vi "linspace_double.vi"(9 "start":dbl format="%0.2f", 10 "end":dbl=1.0 format="%0.2f", 11 "samples":dbl=128.0) -> (3 "Ramp Pattern":dbl[](array[numeric]))   [LabVIEW 2019]
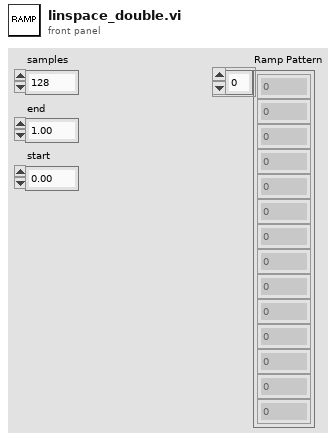
[diagram p1: front panel]
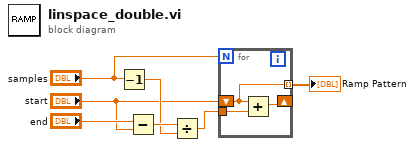
[diagram p0: block diagram]
diagram:
  n1 = Decrement(x="samples") -> (x-1=w6:dbl)
  n2 = Subtract(x="end", y="start") -> (x-y=w7:dbl)
  n3 = Divide(x=w7, y=w6) -> (x/y=w4:dbl)
  n4 = for {
    N: "samples" -> [_]
    shift-right: [w10] -> _
    shift-left: "start" -> [w8]
    tunnel: w4 -> [w9]
    tunnel: [w8] -> w3 mode=indexing
    n5 = Add(x=w8, y=w9) -> (x+y=w10:dbl)
  }
  "Ramp Pattern" <- w3
